vi "CRYPEAQ tConst.vi"(8 "Fss":dbl, 9 "f(fc)":dbl[](array[numeric]) format="%#.6f", 10 "tmin":dbl=0.008, 11 "t100":dbl=0.05) -> (2 "b":dbl[](array[numeric]), 3 "a":dbl[](array[numeric]))   [LabVIEW 2013]
panel:
  out "Waveform Graph":dbl[](graph)
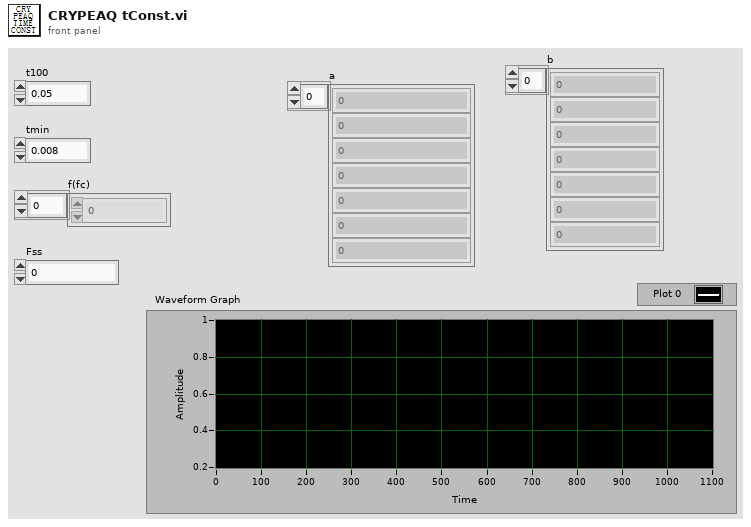
[diagram p1: front panel]
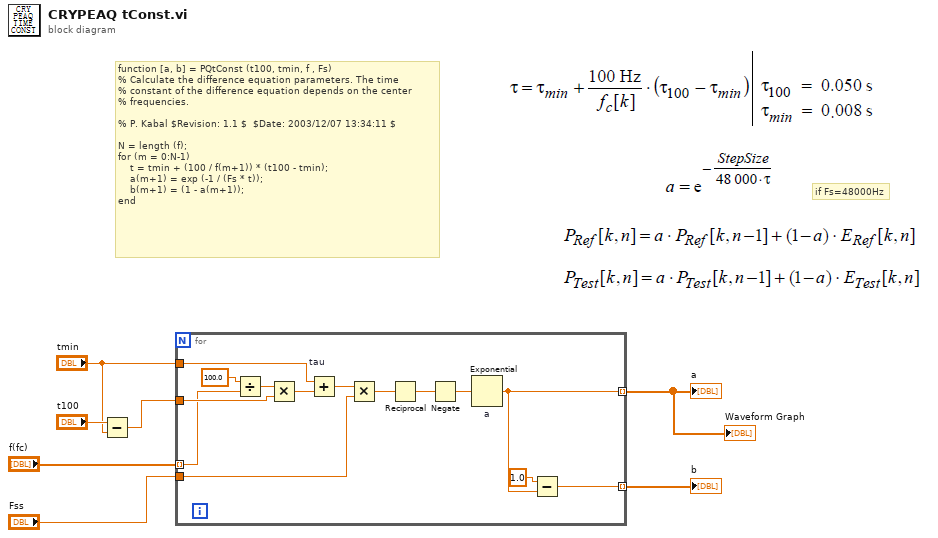
[diagram p0: block diagram]
diagram:
  # "if Fs=48000Hz"
  # "function [a, b] = PQtConst (t100, tmin, f , Fs)\n% Calculate the difference equation parameters. The time\n% constant of the difference equation depends on the center\n% frequencies.\n\n% P. Kabal $Revision: 1.1 $  $Date: 2003/12/07 13:34:11 $\n\nN = length (f);\nfor (m = 0:N-1)\n    t = tmin + (100 / f(m+1)) * (t100 - tmin);\n    a(m+1) = exp (-1 / (Fs * t));\n    b(m+1) = (1 - a(m+1));\nend"
  n1 = Subtract(x="t100", y="tmin") -> (x-y=w4:dbl)
  n2 = for {
    tunnel: "f(fc)" -> [w14] mode=indexing
    tunnel: w4 -> [w16]
    tunnel: "tmin" -> [w15]
    tunnel: [w9] -> w1 mode=indexing
    tunnel: [w8] -> w2 mode=indexing
    tunnel: "Fss" -> [w10]
    n3 = Divide(x=100.0, y=w14) -> (x/y=w18:dbl)
    n4 = Multiply(x=w18, y=w16) -> (x*y=w19:dbl)
    n5 = Add "tau"(x=w15, y=w19) -> (x+y=w13:dbl)
    n6 = Multiply(x=w13, y=w10) -> (x*y=w11:dbl)
    n7 = Reciprocal(x=w11) -> (1/x=w20:dbl)
    n8 = Negate(x=w20) -> (-x=w12:dbl)
    n9 = Exponential "a"(1:w12) -> (0:w9:dbl)
    n10 = Subtract(x=1.0, y=w9) -> (x-y=w8:dbl)
  }
  "b" <- w2
  "a" <- w1
  "Waveform Graph" <- w1
